vi "changeControl.vi"(6 "라벨명(str)":string[](array[string]), 8 "error in":errorcluster caption="에러 입력", 9 "라벨명":string[](array[string]), 10 "기능":enum16{"LOAD", "SAVE"}(ring), 11 "VI 참조":refnum<vi>) -> (0 "error out":errorcluster caption="에러 출력")   [LabVIEW 2018]
uses:
  JKI-JSON-Serialization/src/JKI JSON Serialization.lvlib
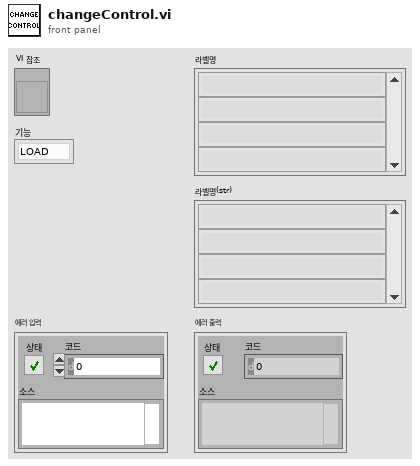
[diagram p1: front panel]
types:
  T1 = enum16{"open", "replace", "create", "open or create", "replace or create", "replace or create with confirmation"}
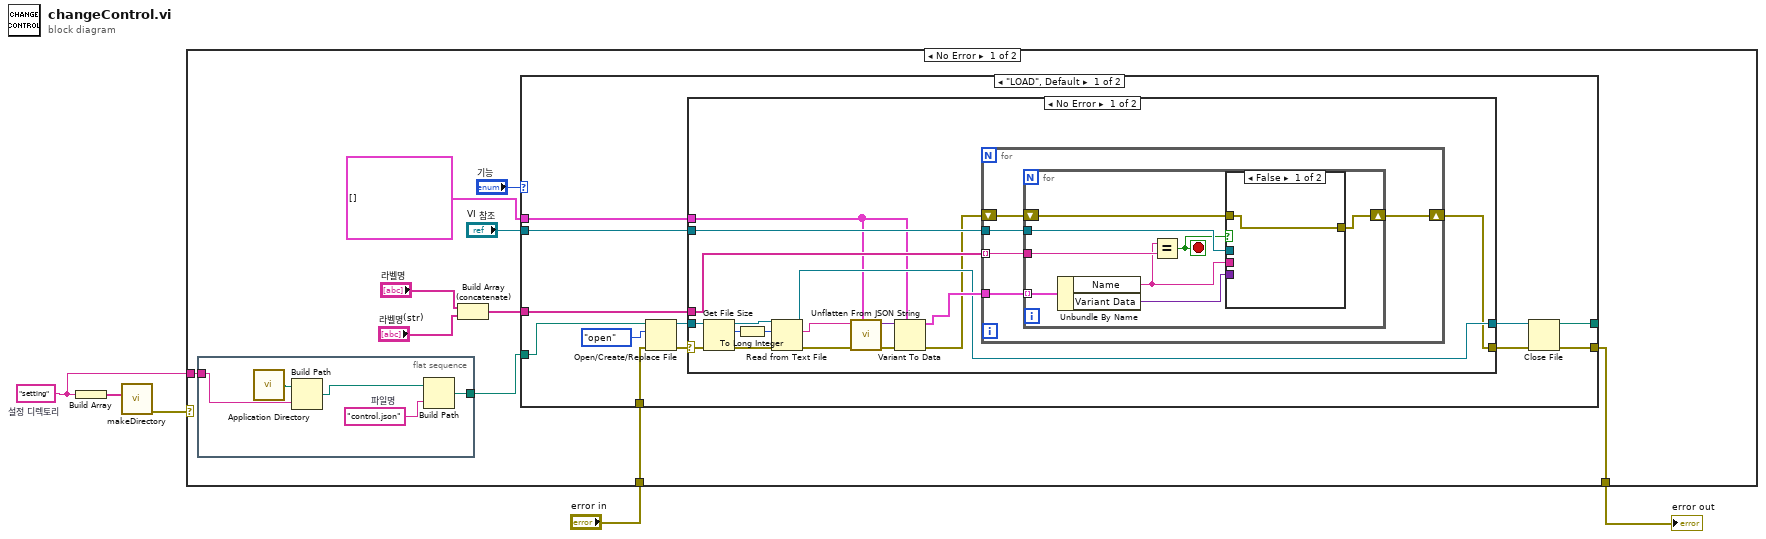
[diagram p0: block diagram]
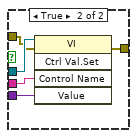
[diagram p2: hidden frame]
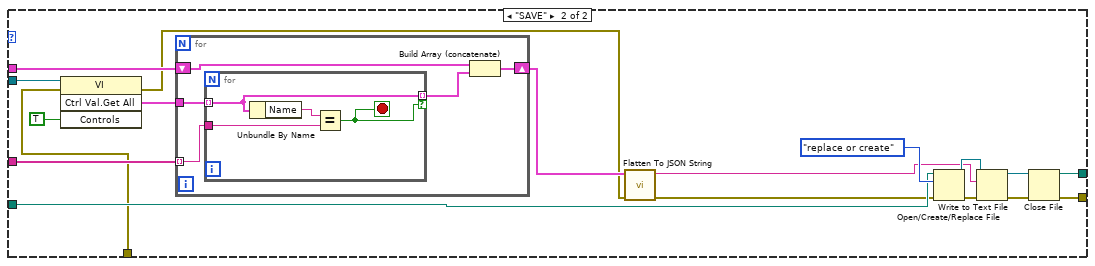
[diagram p4: hidden frame]
diagram:
  w1 = "setting"  # 설정 디렉토리
  n1 = Build Array(w1) -> (w5:string[])
  n2 = call "makeDirectory.vi"("설정 디렉토리"=w5) -> ("error out"=w4:errorcluster)  [unwired: 10 in]
  n3 = case shown="No Error" w4 {
    tunnel: "error in" -> [w8 w98]
    tunnel: [w7 w98] -> w2
    tunnel: w1 -> [w6 _]
    frame No Error {
      n4 = flat-sequence {
        tunnel: [w20] -> w13
        tunnel: w6 -> [w17]
        frame #0 {
          w19 = "control.json"  # 파일명
          n5 = call <vilib>:"Application Directory.vi"() -> ("Application Directory"=w18:path)
          n6 = Build Path(base path=w18, name or relative path=w17) -> (appended path=w16:path)
          n7 = Build Path(base path=w16, name or relative path=w19) -> (appended path=w20:path)
        }
      }
      n8 = Build Array (concatenate)("라벨명", "라벨명(str)") -> (w9:string[])
      n9 = case shown="\"LOAD\", Default" "기능" {
        tunnel: w9 -> [w28 w77]
        tunnel: [w22 w72] -> _
        tunnel: [w21 w71] -> w7
        tunnel: w13 -> [w31 w85]
        tunnel: cluster{"Name":string, "Variant Data":variant}[] [] ("컨트롤 값:모두 얻기") -> [w30 w84]
        tunnel: "VI 참조" -> [w26 w79]
        tunnel: w8 -> [w25 w76]
        frame "LOAD", Default {
          n10 = Open/Create/Replace File(file path (use dialog)=w31, error in=w25, operation (0:open)=T1."open" ("동작(0:open)")) -> (refnum out=w29:refnum<file>, error out=w27:errorcluster)  [unwired: 3 in, 1 out]
          n11 = case shown="No Error" w27 {
            selector: w27 -> [w41 w70]
            tunnel: w30 -> [w37 _]
            tunnel: [w47 w69] -> w24
            tunnel: w29 -> [w43 w69]
            tunnel: w28 -> [w49 _]
            tunnel: [w33 w70] -> w23
            tunnel: w26 -> [w38 _]
            frame No Error {
              n12 = Get File Size(file=w43, error in=w41) -> (refnum out=w42:refnum<file>, size (in bytes)=w44:i64, 0:w40:errorcluster)
              n13 = To Long Integer(number=w44) -> (32bit integer=w39:i32)
              n14 = Read from Text File(file (use dialog)=w42, count=w39, error in=w40) -> (refnum out=w47:refnum<file>, text=w45:string, error out=w46:errorcluster)  [unwired: 1 in, 1 out]
              n15 = call "Unflatten From JSON String.vi"("Type and Defaults"=w37, "error in (no error)"=w46, "JSON String"=w45) -> ("error out"=w35:errorcluster, "Variant"=w36:variant)  [unwired: 7 in]
              n16 = Variant To Data(error in=w35, type=w37, Variant=w36) -> (data=w48:cluster{"Name":string, "Variant Data":variant}[], error out=w34:errorcluster)
              n17 = for {
                tunnel: w48 -> [w54]
                tunnel: w49 -> [w53] mode=indexing
                tunnel: w38 -> [w52]
                shift-right: [w50] -> w33
                shift-left: w34 -> [w51]
                n18 = for {
                  tunnel: w54 -> [w62] mode=indexing
                  tunnel: w53 -> [w61]
                  tunnel: w52 -> [w58]
                  shift-right: [w55] -> w50
                  shift-left: w51 -> [w56]
                  stop <- w57 stop-if-true
                  n19 = Unbundle By Name(w62) -> ("Name"=w60:string, "Variant Data"=w59:variant)
                  n20 = Equal?(x=w60, y=w61) -> (x = y?=w57:bool)
                  n21 = case shown="False" w57 {
                    tunnel: w60 -> [_ w68]
                    tunnel: w59 -> [_ w67]
                    tunnel: w58 -> [_ w66]
                    tunnel: w56 -> [w63 w65]
                    tunnel: [w63 w64] -> w55
                    frame False {
                    }
                    frame True {
                      n22 = invoke class="VI" method="Ctrl Val.Set"(reference=w66, error in=w65, "Control Name"=w68, "Value"=w67) -> (error out=w64:errorcluster)  [unwired: 1 in, 4 out]
                    }
                  }
                }
              }
            }
            frame Error {
            }
          }
          n23 = Close File(refnum=w24, error in=w23) -> (path=w22:path, error out=w21:errorcluster)
        }
        frame "SAVE" {
          n24 = invoke class="VI" method="Ctrl Val.Get All"(reference=w79, error in=w76, "Controls"=TRUE ("컨트롤")) -> (error out=w75:errorcluster, "Get All Control Values Variant"=w82:cluster{"Name":string, "Variant Data":variant}[])  [unwired: 1 in, 2 out]
          n25 = for {
            tunnel: w82 -> [w93]
            tunnel: w77 -> [w92] mode=indexing
            shift-right: [w91] -> w78
            shift-left: w84 -> [w90]
            n26 = for {
              tunnel: w93 -> [w94] mode=indexing
              tunnel: w92 -> [w96]
              tunnel: [w94] -> w89 mode=indexing if=w95
              stop <- w95 stop-if-true
              n27 = Unbundle By Name(w94) -> ("Name"=w97:string)
              n28 = Equal?(x=w97, y=w96) -> (x = y?=w95:bool)
            }
            n29 = Build Array (concatenate)(w90, w89) -> (w91:cluster{"Name":string, "Variant Data":variant}[])
          }
          n30 = call "Flatten To JSON String.vi"("error in (no error)"=w75, "Variant"=w78) -> ("error out"=w80:errorcluster, "JSON String"=w81:string)  [unwired: 8 in]
          n31 = Open/Create/Replace File(file path (use dialog)=w85, error in=w80, operation (0:open)=T1."replace or create" ("동작(0:open)")) -> (refnum out=w87:refnum<file>, error out=w88:errorcluster)  [unwired: 3 in, 1 out]
          n32 = Write to Text File(file (use dialog)=w87, text=w81, error in=w88) -> (refnum out=w74:refnum<file>, error out=w73:errorcluster)  [unwired: 1 in, 1 out]
          n33 = Close File(refnum=w74, error in=w73) -> (path=w72:path, error out=w71:errorcluster)
        }
      }
    }
    frame Error {
    }
  }
  "error out" <- w2
